vi "Thermi(ABC).vi"(8 "Temp":dbl[](array[numeric])=[25.0, 75.0, 125.0], 11 "Thermistor":dbl[](array[numeric])=[10000.0, 1897.904, 546.7892]) -> (1 "γ":dbl, 2 "β":dbl format="%#_6e", 3 "α":dbl format="%#_6e")   [LabVIEW 2012]
doc: "功能：\n\n由于不同型号的热敏电阻，参数A B C的差别比较大，该VI通过给定三组温度和阻值的试验数据，自动解三元一次方程组，求取系数A B C的值。\n\n默认值为NTC的三组数据。"
uses:
  <vilib>/Analysis/7linalg.llb/Solve Linear Equations (single right hand).vi
  <vilib>/Analysis/7linalg.llb/Solve Linear Eqs (General).vi
  <vilib>/Analysis/7linalg.llb/Solve Linear Eqs (Gen, single right hand).vi
  <vilib>/Analysis/NI_AALPro.lvlib
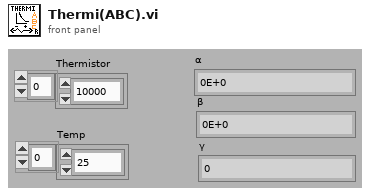
[diagram p1: front panel]
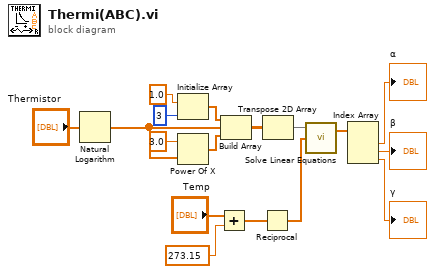
[diagram p0: block diagram]
diagram:
  n1 = Natural Logarithm(1:"Thermistor") -> (0:w11:dbl[])
  n2 = Initialize Array(1.0 ("元素"), 3 ("维数大小")) -> (w12:dbl[])
  n3 = Power Of X(1:w11, 2:3.0 ("y")) -> (0:w10:dbl[])
  n4 = Add(x="Temp", y=273.15) -> (x+y=w15:dbl[])
  n5 = Build Array(w12, w11, w10) -> (w5:dbl[][])
  n6 = Reciprocal(x=w15) -> (1/x=w8:dbl[])
  n7 = Transpose 2D Array(2D array=w5) -> (transposed array=w9:dbl[][])
  n8 = call-poly <vilib>:"Solve Linear Equations.vi"("Known Vector"=w8, "Input Matrix"=w9) -> ("Solution Vector"=w4:dbl[])  [unwired: 1 in, 1 out]
  n9 = Index Array(array=w4) -> (element #1=→"α":dbl, element #2=→"β":dbl, element #3=→"γ":dbl)  [unwired: 3 in]
